vi "SeCrTs-Data reader from shared variable.vi"(0 "Config":T1, 1 "Start/Stop Log":bool[](array[boolean]), 2 "Log Name":string, 3 "C/NC":bool, 4 "Log min":dbl, 5 "error IO":errorcluster, 7 "empty?":bool) -> (19 "error out":errorcluster)   [LabVIEW 2022 SP3]
uses:
  91644d88-8a3a-46f6-9314-183f243c8ec6.vi
  3d41d14a-1e81-4e0e-8a5a-4fdd32b6dd05.vi
  Globals/SeCrTS-DD globals.vi
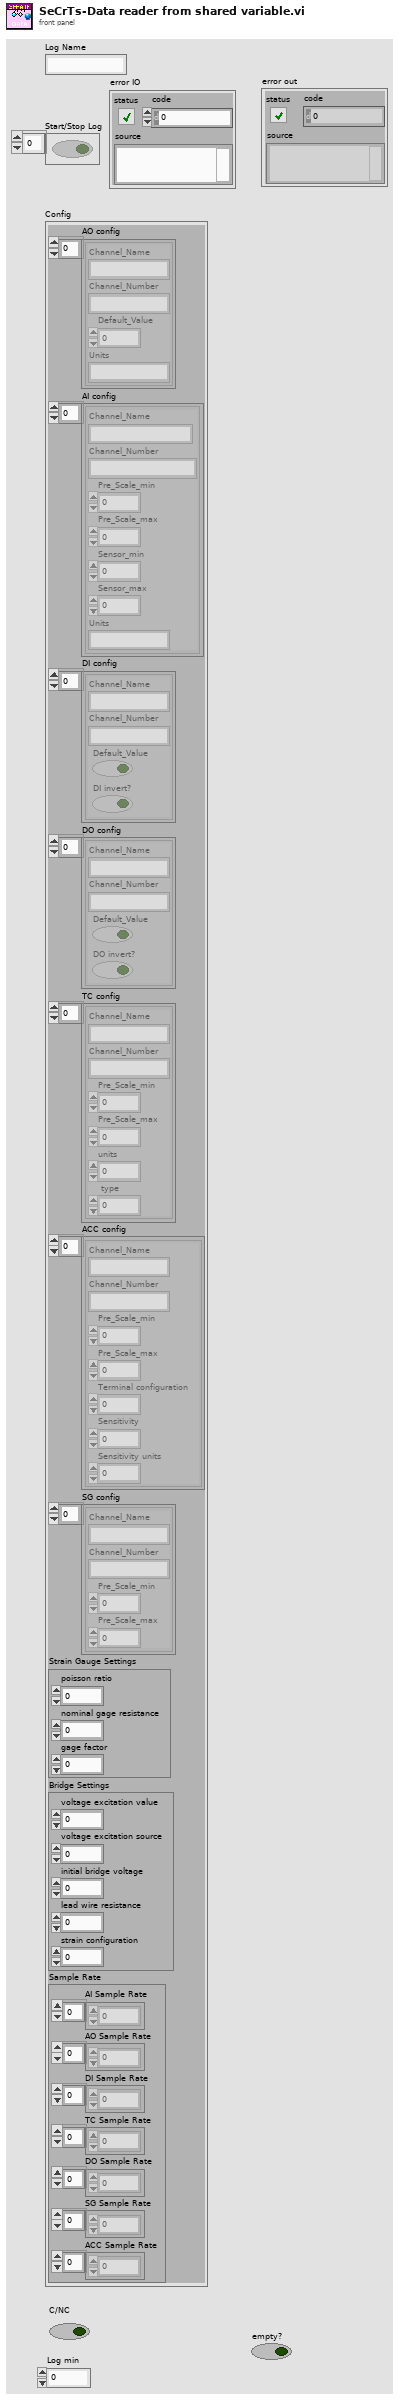
[diagram p1: front panel]
types:
  T1 = cluster{"AO config":cluster{"Channel_Name":string, "Channel_Number":string, "Default_Value":dbl, "Units":string}[], "AI config":cluster{"Channel_Name":string, "Channel_Number":string, "Pre_Scale_min":dbl, "Pre_Scale_max":dbl, "Sensor_min":dbl, "Sensor_max":dbl, "Units":string}[], "DI config":cluster{"Channel_Name":string, "Channel_Number":string, "Default_Value":bool, "DI invert?":bool}[], "DO config":cluster{"Channel_Name":string, "Channel_Number":string, "Default_Value":bool, "DO invert?":bool}[], "TC config":cluster{"Channel_Name":string, "Channel_Number":string, "Pre_Scale_min":dbl, "Pre_Scale_max":dbl, "units":i32, " type":i32}[], "ACC config":cluster{"Channel_Name":string, "Channel_Number":string, "Pre_Scale_min":dbl, "Pre_Scale_max":dbl, "Terminal configuration":i32, "Sensitivity":dbl, "Sensitivity units":i32}[], "SG config":cluster{"Channel_Name":string, "Channel_Number":string, "Pre_Scale_min":dbl, "Pre_Scale_max":dbl}[], "Strain Gauge Settings":cluster{"poisson ratio":dbl, "nominal gage resistance":dbl, "gage factor":dbl}, "Bridge Settings":cluster{"voltage excitation value":dbl, "voltage excitation source":i32, "initial bridge voltage":dbl, "lead wire resistance":dbl, "strain configuration":i32}, "Sample Rate":cluster{"AI Sample Rate":dbl[], "AO Sample Rate":dbl[], "DI Sample Rate":dbl[], "TC Sample Rate":dbl[], "DO Sample Rate":dbl[], "SG Sample Rate":dbl[], "ACC Sample Rate":dbl[]}}
  T2 = cluster{"Channel names":cluster{"AI_C_Data P":string[], "AI_V_Data P":string[], "AO_Data P":string[], "DO_Data P":string[], "ACC_Data P":string[], "TC Data P":string[], "Drive_A_C":string[], "Drive_A_D":string[], "AI_C_Data S":string[], "DO_Data S":string[]}, "DI Names":cluster{"Di P":string[], "Di S":string[]}}
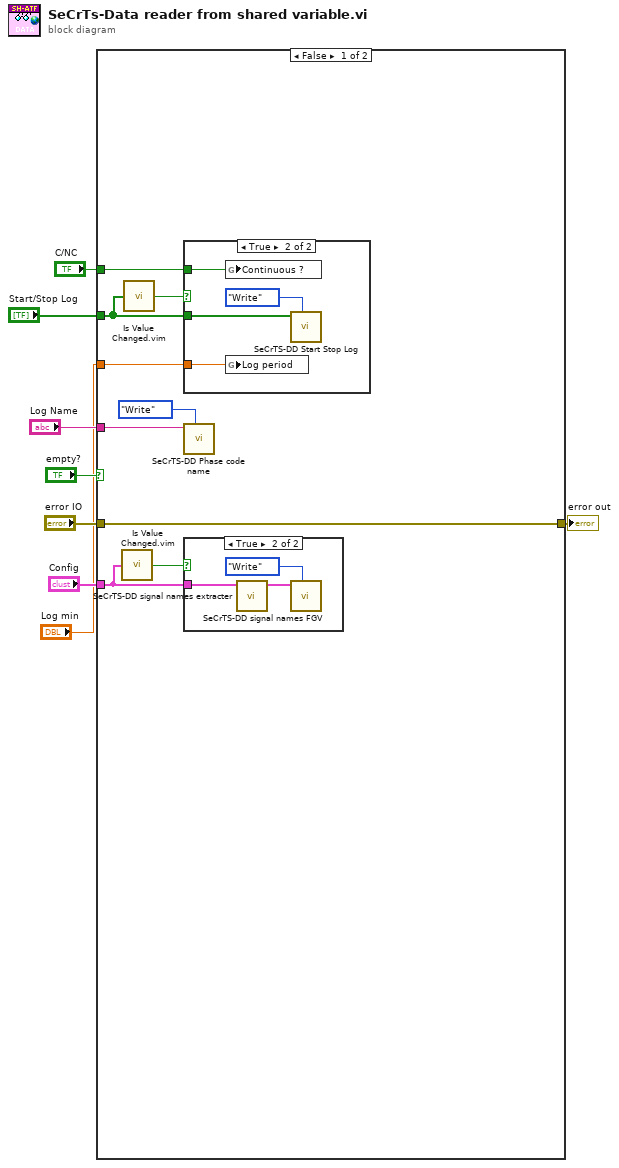
[diagram p0: block diagram]
diagram:
  n1 = case shown="False" "empty?" {
    tunnel: "Log Name" -> [w16 _]
    tunnel: "Config" -> [w13 _]
    tunnel: "Start/Stop Log" -> [w12 _]
    tunnel: "error IO" -> [w11 w25]
    tunnel: [w11 w25] -> w3
    tunnel: "C/NC" -> [w10 _]
    tunnel: "Log min" -> [w9 _]
    frame False {
      n2 = call "Is Value Changed.vim"("value"=w13) -> ("changed or first call?"=w15:bool)
      n3 = call "Is Value Changed.vim"("value"=w12) -> ("changed or first call?"=w14:bool)
      n4 = case shown="True" w14 {
        tunnel: w12 -> [_ w20]
        tunnel: w10 -> [_ w18]
        tunnel: w9 -> [_ w19]
        frame False {
        }
        frame True {
          n5 = global write "SeCrTS-DD globals.vi" "Continuous ?"(w18) -> ()
          n6 = global write "SeCrTS-DD globals.vi" "Log period"(w19) -> ()
          n7 = call "SeCrTS-DD Start Stop Log.vi"("Enum"=enum16{"Read", "Write"}."Write", "Start Stop log"=w20) -> ()  [unwired: 8 in, 2 out]
        }
      }
      n8 = call "SeCrTS-DD Phase code name.vi"("Enum"=enum16{"Read", "Write"}."Write", "Phase code W"=w16) -> ()  [unwired: 8 in, 2 out]
      n9 = case shown="True" w15 {
        tunnel: w13 -> [_ w24]
        frame False {
        }
        frame True {
          n10 = call "SeCrTS-DD signal names extracter.vi"("input cluster"=w24) -> ("Signal names"=w23:T2)  [unwired: 10 in]
          n11 = call "SeCrTS-DD signal names FGV.vi"("Enum"=enum16{"Read", "Write"}."Write", "Signal names"=w23) -> ()  [unwired: 8 in, 2 out]
        }
      }
    }
    frame True {
    }
  }
  "error out" <- w3
